vi "OnCommand(SingleObject).vi"(10 "Command ID":string, 11 "Object":T1) -> ()   [LabVIEW 2017]
uses:
  <resource>/Framework/Providers/API/ItemRef.ctl
  <vilib>/Utility/miscctls.llb/LVRectTypeDef.ctl
  user.lib/_NEVSTOP/Communicable State Machine(CSM)/_xnode/csm_tool/_xnode_csm_tool_support/CSM DebugTool Dialog.lvlib
  user.lib/_NEVSTOP/Communicable State Machine(CSM)/_Shared/CSM Shared.lvlib
panel:
  # "PROJFILE_TRIGGER_BUILDSYSTEM\nPROJFILE_TRIGGER_TESTSYSTEM"
  # "VFOLDER_TRIGGER_BUILDSYSTEM\nVFOLDER_TRIGGER_TESTSYSTEM"
  # "ToolProviders_SCANTOOLS\nToolProviders_xxxxx"
  # "PINMAPFILE_xxxxxx"
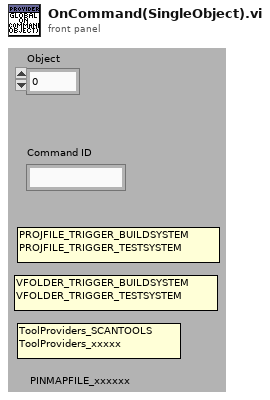
[diagram p1: front panel]
types:
  T1 = typedef "ItemRef.ctl" = u64
  T2 = typedef "LVRectTypeDef.ctl" = cluster{"Left":i16, "Top":i16, "Right":i16, "Bottom":i16}
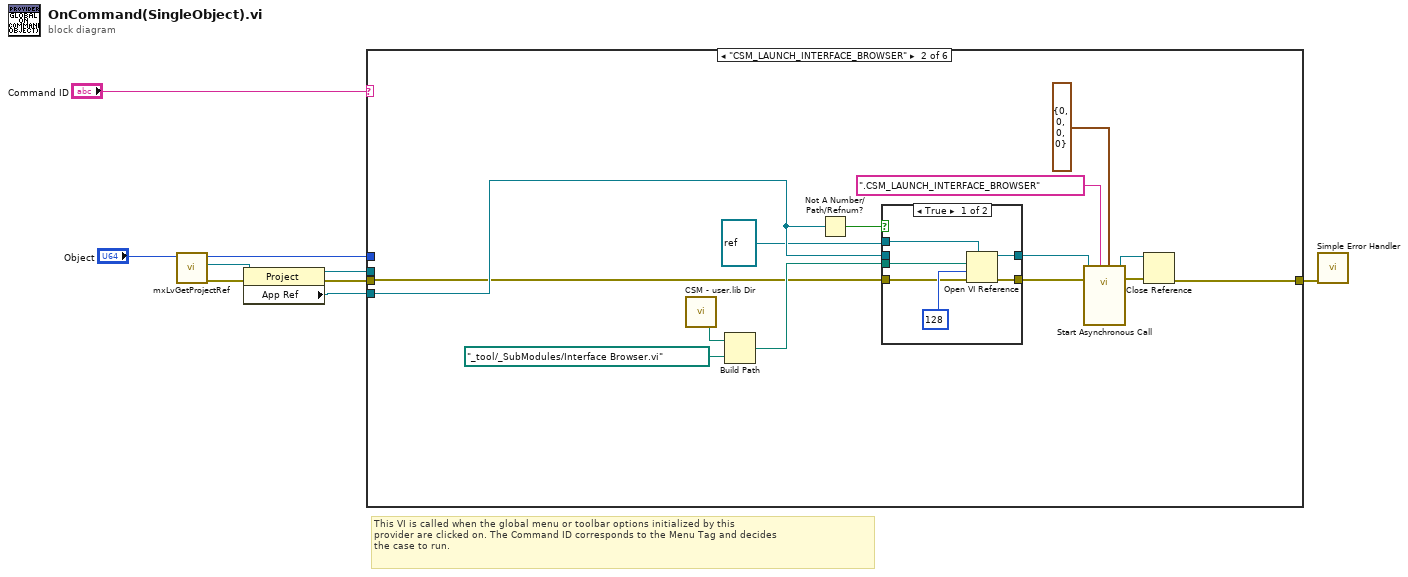
[diagram p0: block diagram]
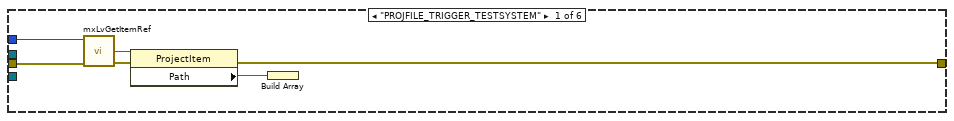
[diagram p2: hidden frame]
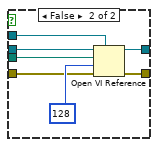
[diagram p3: hidden frame]
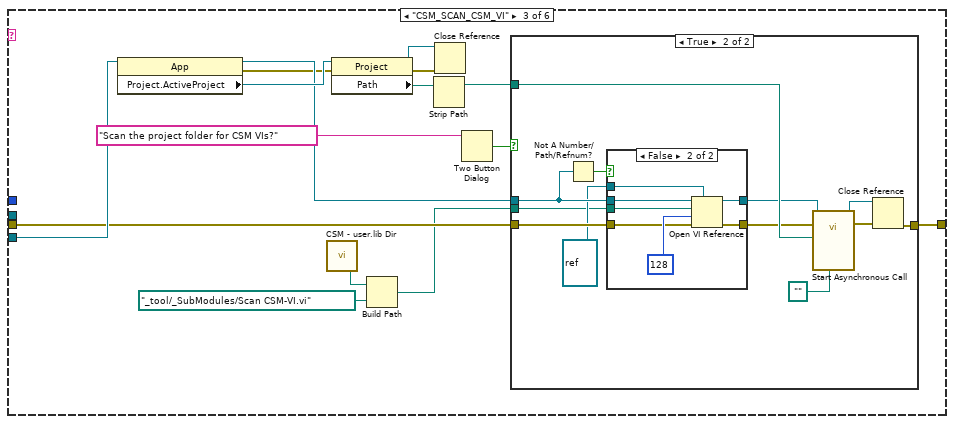
[diagram p4: hidden frame]
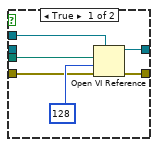
[diagram p6: hidden frame]
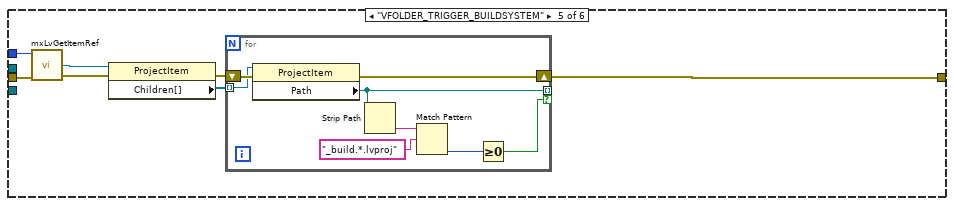
[diagram p8: hidden frame]
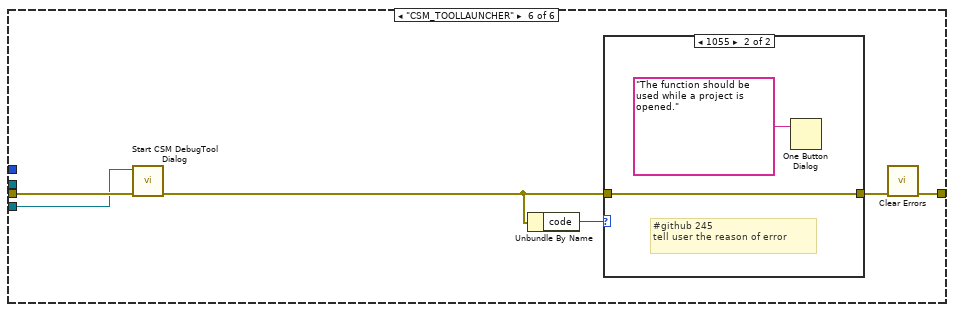
[diagram p9: hidden frame]
diagram:
  # "This VI is called when the global menu or toolbar options initialized by this \nprovider are clicked on. The Command ID corresponds to the Menu Tag and decides\nthe case to run."
  n1 = call <resource>:"mxLvGetProjectRef.vi"("Item"="Object") -> ("error out"=w8:errorcluster, "Project Refnum"=w7:refnum<vi>, "Item"=w5:T1)  [unwired: 8 in]
  n2 = property class="Project"(reference=w7, error in=w8) -> (reference out=w3:refnum<vi>, error out=w4:errorcluster, "App Ref"=w2:refnum<vi>)
  n3 = case shown="\"CSM_LAUNCH_INTERFACE_BROWSER\"" "Command ID" {
    tunnel: [w11 w22 w48 w84 w87 w100] -> w1
    tunnel: w5 -> [w13 _ _ _ w91 _]
    tunnel: w4 -> [w12 w19 w50 w84 w90 w104]
    tunnel: w2 -> [_ w23 w51 _ _ w103]
    tunnel: w3 -> [_ _ _ _ _ _]
    frame "PROJFILE_TRIGGER_TESTSYSTEM" {
      n4 = call <resource>:"mxLvGetItemRef.vi"("Item"=w13, "error in"=w12) -> ("Item Refnum"=w15:refnum<vi>, "error out"=w14:errorcluster)  [unwired: 1 out]
      n5 = property class="ProjectItem"(reference=w15, error in=w14) -> (error out=w11:errorcluster, "Path"=w10:path)  [unwired: 1 out]
      n6 = Build Array(w10) -> ()  [unwired: 1 out]
    }
    frame "CSM_LAUNCH_INTERFACE_BROWSER" {
      n7 = call "CSM - user.lib Dir.vi"() -> ("csm_user.lib_dir"=w21:path)  [unwired: 2 in, 1 out]
      n8 = Build Path(base path=w21, name or relative path=path "_tool/_SubModules/Interface Browser.vi" ("execute path")) -> (appended path=w20:path)
      n9 = Not A Number/Path/Refnum?(number/path/refnum=w23) -> (NaN/Path/Refnum?=w24:bool)
      n10 = case shown="True" w24 {
        tunnel: refnum<vi> refnum -> [w34 w41]
        tunnel: [w33 w40] -> w26
        tunnel: w19 -> [w32 w39]
        tunnel: w20 -> [w31 w38]
        tunnel: [w30 w37] -> w25
        tunnel: w23 -> [_ w36]
        frame True {
          n11 = Open VI Reference(type specifier VI Refnum (for type only)=w34, vi path=w31, options=128, error in (no error)=w32) -> (vi reference=w33:refnum<vi>, error out=w30:errorcluster)  [unwired: 2 in]
        }
        frame False {
          n12 = Open VI Reference(type specifier VI Refnum (for type only)=w41, application reference (local)=w36, vi path=w38, options=128, error in (no error)=w39) -> (vi reference=w40:refnum<vi>, error out=w37:errorcluster)  [unwired: 1 in]
        }
      }
      n13 = call-by-ref "Start Asynchronous Call"(reference=w26, error in=w25, "Caller Window Bounds"=T2 {"Left"=0, "Top"=0, "Right"=0, "Bottom"=0}, "Name (\"\" to Use Uuid)"=".CSM_LAUNCH_INTERFACE_BROWSER" ("Name (\"\" to Use Uuid)")) -> (reference out=w28:refnum<vi>, error out=w27:errorcluster)  [unwired: 10 in]
      n14 = Close Reference(reference=w28, error in (no error)=w27) -> (error out=w22:errorcluster)
    }
    frame "CSM_SCAN_CSM_VI" {
      n15 = property class="App"(reference=w51) -> (reference out=w52:refnum<vi>, error out=w46:errorcluster, "Project.ActiveProject"=w53:refnum<vi>)  [unwired: 1 in]
      n16 = call "CSM - user.lib Dir.vi"() -> ("csm_user.lib_dir"=w56:path)  [unwired: 2 in, 1 out]
      n17 = property class="Project"(reference=w53, error in=w46) -> (reference out=w45:refnum<vi>, error out=w47:errorcluster, "Path"=w54:path)
      n18 = Build Path(base path=w56, name or relative path=path "_tool/_SubModules/Scan CSM-VI.vi" ("execute path")) -> (appended path=w49:path)
      n19 = Strip Path(path=w54) -> (stripped path=w55:path)  [unwired: 1 out]
      n20 = Close Reference(reference=w45, error in (no error)=w47) -> ()  [unwired: 1 out]
      n21 = Two Button Dialog(message="Scan the project folder for CSM VIs?") -> (T button?=w44:bool)  [unwired: 2 in]
      n22 = case shown="True" w44 {
        tunnel: w55 -> [_ w70]
        tunnel: w52 -> [_ w69]
        tunnel: w50 -> [w58 w62]
        tunnel: w49 -> [_ w60]
        tunnel: [w58 w59] -> w48
        frame False {
        }
        frame True {
          n23 = Not A Number/Path/Refnum?(number/path/refnum=w69) -> (NaN/Path/Refnum?=w68:bool)
          n24 = case shown="False" w68 {
            tunnel: refnum<vi> refnum -> [w75 w82]
            tunnel: [w74 w81] -> w66
            tunnel: w62 -> [w73 w80]
            tunnel: w60 -> [w72 w79]
            tunnel: [w71 w78] -> w67
            tunnel: w69 -> [_ w77]
            frame True {
              n25 = Open VI Reference(type specifier VI Refnum (for type only)=w75, vi path=w72, options=128, error in (no error)=w73) -> (vi reference=w74:refnum<vi>, error out=w71:errorcluster)  [unwired: 2 in]
            }
            frame False {
              n26 = Open VI Reference(type specifier VI Refnum (for type only)=w82, application reference (local)=w77, vi path=w79, options=128, error in (no error)=w80) -> (vi reference=w81:refnum<vi>, error out=w78:errorcluster)  [unwired: 1 in]
            }
          }
          n27 = call-by-ref "Start Asynchronous Call"(reference=w66, error in=w67, "Config Path"=path "", "root"=w70) -> (reference out=w64:refnum<vi>, error out=w65:errorcluster)  [unwired: 9 in, 1 out]
          n28 = Close Reference(reference=w64, error in (no error)=w65) -> (error out=w59:errorcluster)
        }
      }
    }
    frame Default {
    }
    frame "VFOLDER_TRIGGER_BUILDSYSTEM" {
      n29 = call <resource>:"mxLvGetItemRef.vi"("Item"=w91, "error in"=w90) -> ("Item Refnum"=w85:refnum<vi>, "error out"=w86:errorcluster)  [unwired: 1 out]
      n30 = property class="ProjectItem"(reference=w85, error in=w86) -> (error out=w88:errorcluster, "Children[]"=w89:refnum<vi>[])  [unwired: 1 out]
      n31 = for {
        shift-right: [w98] -> w87
        shift-left: w88 -> [w99]
        tunnel: w89 -> [w97] mode=indexing
        tunnel: [w96] -> _ mode=indexing if=w92
        n32 = property class="ProjectItem"(reference=w97, error in=w99) -> (error out=w98:errorcluster, "Path"=w96:path)  [unwired: 1 out]
        n33 = Strip Path(path=w96) -> (name=w93:string)  [unwired: 1 out]
        n34 = Match Pattern(string=w93, regular expression="_build.*.lvproj") -> (offset past match=w95:i32)  [unwired: 1 in, 3 out]
        n35 = Greater Or Equal To 0?(x=w95) -> (x >= 0?=w92:bool)
      }
    }
    frame "CSM_TOOLLAUNCHER" {
      n36 = call "Start CSM DebugTool Dialog.vi"("error in (no error)"=w104, "Application In"=w103) -> ("error out"=w102:errorcluster)  [unwired: 9 in]
      n37 = Unbundle By Name(w102) -> ("code"=w101:i32)
      n38 = case shown="1055" w101 {
        tunnel: [w106 w108] -> w105
        tunnel: w102 -> [w106 w108]
        frame 0, Default {
        }
        frame 1055 {
          # "#github 245\ntell user the reason of error"
          n39 = One Button Dialog(message="The function should be used while a project is opened.") -> ()  [unwired: 1 in, 1 out]
        }
      }
      n40 = call <vilib>:"Clear Errors.vi"("error in (no error)"=w105) -> ("error out"=w100:errorcluster)  [unwired: 5 in, 1 out]
    }
  }
  n41 = call <vilib>:"Simple Error Handler.vi"("error in (no error)"=w1) -> ()  [unwired: 4 in, 5 out]
